vi "Unmarshal.vi"(8 "error in (no error)":errorcluster, 10 "Buffer":u8[](array[numeric]), 11 "int32 in":refnum<class "int64.lvclass">) -> (0 "error out":errorcluster, 2 "Buffer Count":i32=8, 3 "int32 out":refnum<class "int64.lvclass">)   [LabVIEW 2020, in "Protobuf RAW.lvlib" / "int64.lvclass"]
uses:
  int64.lvclass
  int64.lvclass/int64.ctl
  Protobuf RAW.lvlib
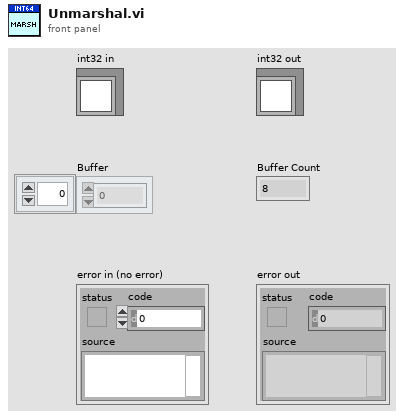
[diagram p1: front panel]
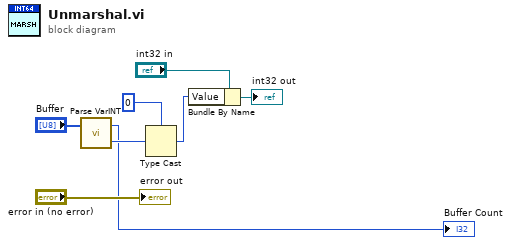
[diagram p0: block diagram]
diagram:
  n1 = call "Parse VarINT.vi"("Buffer"="Buffer") -> ("Numeric"=w4:u64, "Bytes"=→"Buffer Count":i32)  [unwired: 1 in]
  n2 = Type Cast(type=i64 0 ("Numeric"), x=w4) -> (*(type *) &x=w3:i64)
  n3 = Bundle By Name(cluster="int32 in", "Value"=w3) -> (→"int32 out":refnum<class "int64.lvclass">)
  "error out" <- "error in (no error)"
